vi "Script Empty System Definition.vi"(8 "error in":errorcluster, 11 "System Definition Name":string) -> (0 "error out":errorcluster, 3 "System Definition Path":path)   [LabVIEW 2020]
doc: "setUp runs prior to the test method during test execution. Use this method to initialize any object data required by your tests."
uses:
  NationalInstruments.VeriStand.SystemDefinitionAPI
  niveristand-custom-device-testing-tools/VeriStandTestUtilities/VeriStandTestUtilities.lvlib
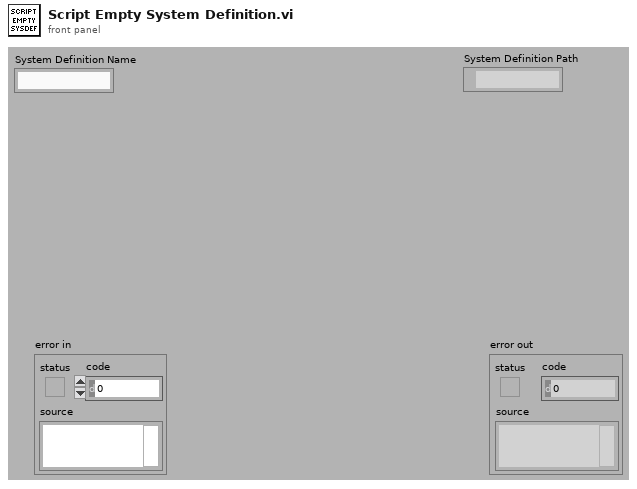
[diagram p1: front panel]
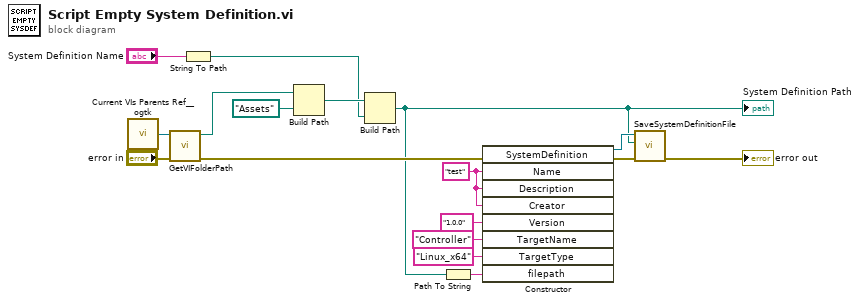
[diagram p0: block diagram]
diagram:
  w12 = "test" ("Name")
  n1 = call <userlib>:"Current VIs Parents Ref__ogtk.vi"() -> ("Calling VI's Reference"=w17:refnum<vi>)  [unwired: 2 in]
  n2 = call "GetVIFolderPath.vi"("error in (no error)"="error in", "VI Reference in"=w17) -> ("error out"=w8:errorcluster, "VI Folder Path out"=w15:path)  [unwired: 8 in]
  n3 = String To Path(string="System Definition Name") -> (path=w1:path)
  n4 = Build Path(base path=w15, name or relative path=path "Assets" ("Absolute or Relative Path")) -> (appended path=w7:path)
  n5 = Build Path(base path=w7, name or relative path=w1) -> (appended path=w4:path)
  "System Definition Path" <- w4
  n6 = Path To String(path=w4) -> (string=w13:string)
  n7 = constructor class="SystemDefinition"(error in=w8, "Name"=w12, "Description"=w12, "Creator"=w12, "Version"="1.0.0", "TargetName"="Controller", "TargetType"="Linux_x64", "filepath"=w13) -> (reference out=w5:refnum<k24>, error out=w6:errorcluster)  [unwired: 2 in, 8 out]
  n8 = call "SaveSystemDefinitionFile.vi"("error in (no error)"=w6, "System Definition File in"=w4, "System Definition Reference in"=w5) -> ("error out"=→"error out":errorcluster)  [unwired: 7 in, 1 out]
